vi "Build Command.vi"(8 "error in":errorcluster, 9 "Input Value":string, 10 "Commands":T1, 11 "ESM303 in":refnum<class "ESM303.lvclass">) -> (0 "error out":errorcluster, 1 "Response Expected?":bool, 2 "Command":string, 3 "ESM303 out":refnum<class "ESM303.lvclass">)   [LabVIEW 2018, in "ESM303.lvlib" / "ESM303.lvclass"]
uses:
  ESM303.lvclass
  builds/Force Test Stand.lvlibp/Custom Controls/Commands.ctl
  <vilib>/regexp/Match Regular Expression.xnode
  builds/Force Test Stand.lvlibp/Force Test Stand.lvclass
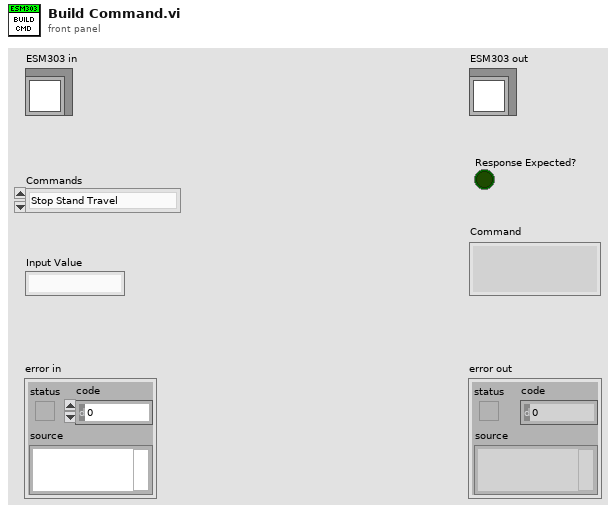
[diagram p1: front panel]
types:
  T1 = typedef "Force Test Stand.lvlibp/Force Test Stand.lvclass/Commands.ctl" = enum16{"Stop Stand Travel", "Start Travel Down (Left)", "Start Travel Up (Right)", "Get Travel Upper Limit", "Get Travel Lower Limit", "Set Travel Upper Limit", "Set Travel Lower Limit", "Get Travel Value", "Set Travel Units (mm)", "Set Travel Units (in)", "Reset Travel to Zero", "Get Speed ", "Set Speed", "Set Speed to Min", "Set Speed to Max", "Get Force Value", "Get Force Units", "Set Force Units (lbF)", "Get Stand Status", "Set Cycle Mode", "Set Limit Mode", "Set Manual Mode", "Set No. Cycles", "Get Travel/Force Values", "Get Completed Cycles", "Get Cycles Setpoint", "Reset Cycles Counter", "Zero Force Gauge", "Set Force Upper Limit", "Set Force Lower Limit", "Get Travel Units", "Get Speed Units", "Default", "Set Force Units (N)", "Set Force Units (kgF)", "Set Force Units (ozF)", "Set Force Units (gF)", "Set Force Real Time Mode", "Set Force Peak Tension Mode", "Set Force Peak Compression Mode", "Set Force High Set-Point", "Set Force Low Set-Point", "Gauge Transmit with Units", "Gauge Transmit w/o Units", "Get Peak Compression Force", "Get Peak Tension Force", "Get Real Time Force", "Disable Force High Limit", "Disable Force Low Limit", "Send Speed Setting to Stand"}
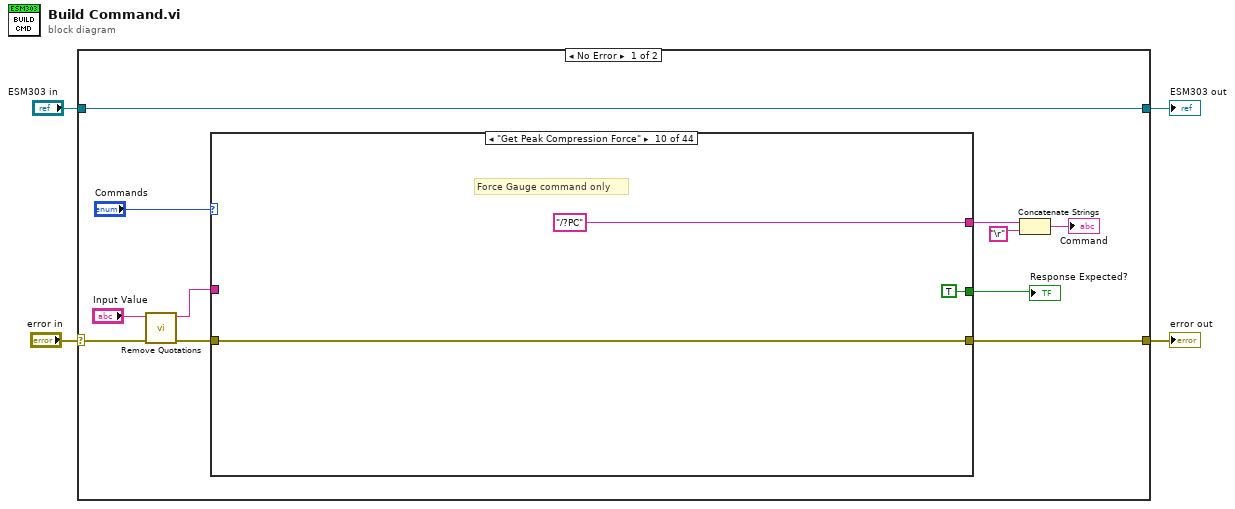
[diagram p0: block diagram]
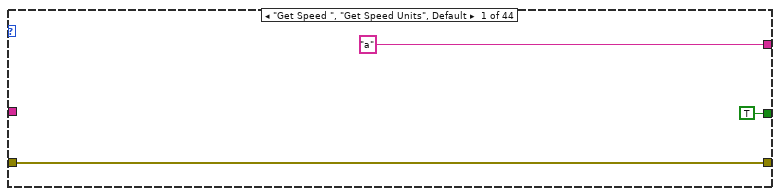
[diagram p2: hidden frame]
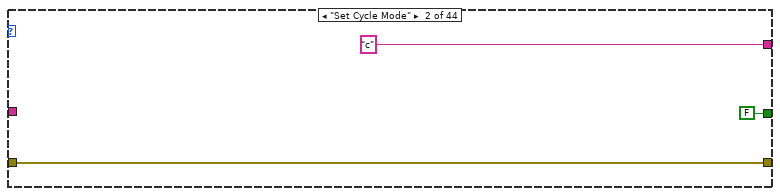
[diagram p3: hidden frame]
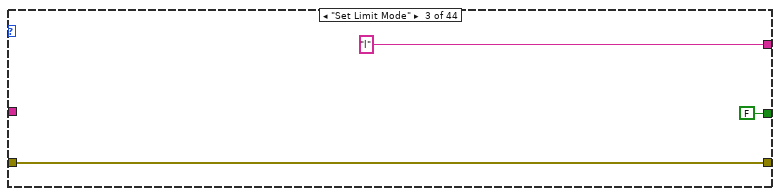
[diagram p4: hidden frame]
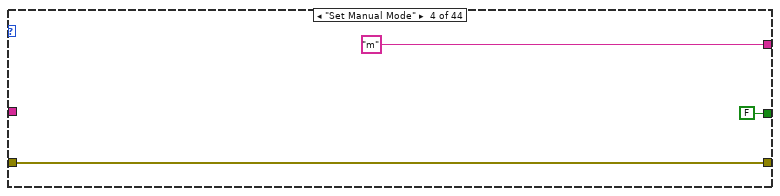
[diagram p5: hidden frame]
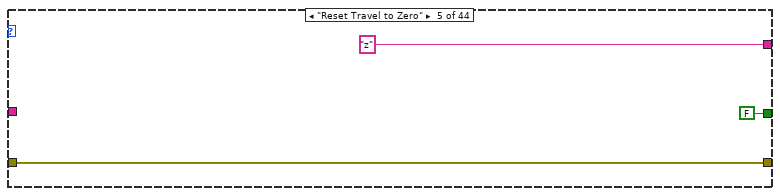
[diagram p6: hidden frame]
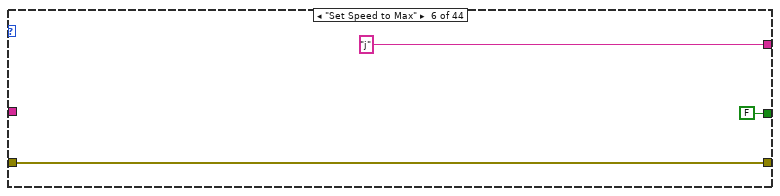
[diagram p7: hidden frame]
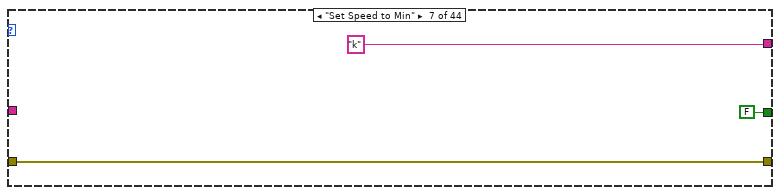
[diagram p8: hidden frame]
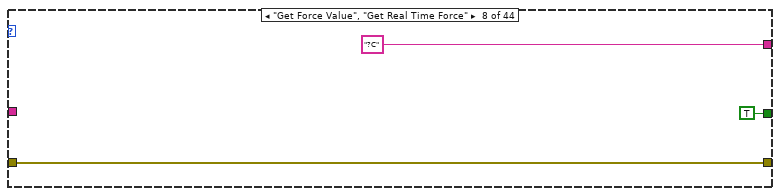
[diagram p9: hidden frame]
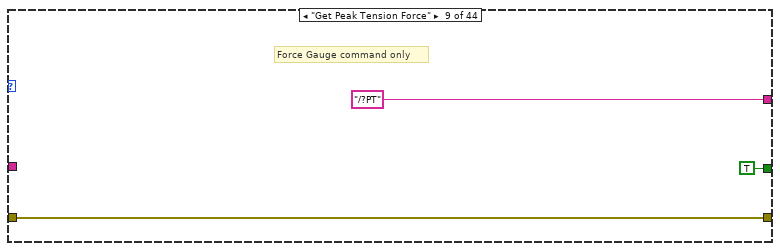
[diagram p10: hidden frame]
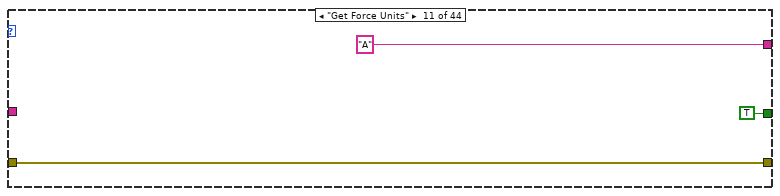
[diagram p11: hidden frame]
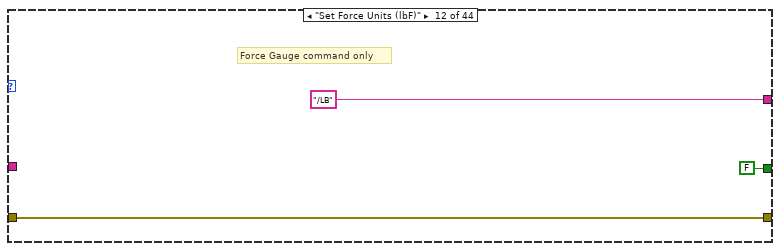
[diagram p12: hidden frame]
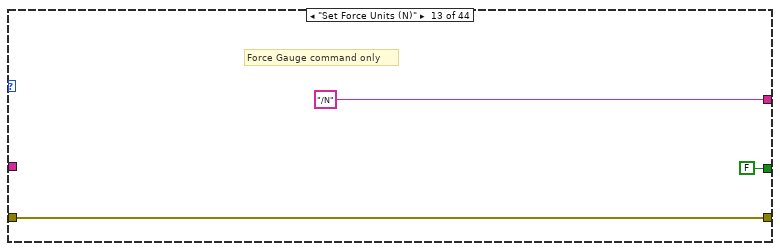
[diagram p13: hidden frame]
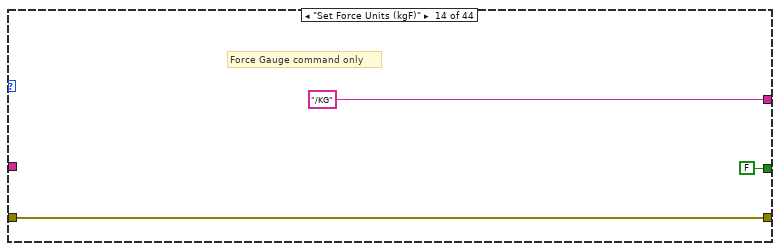
[diagram p14: hidden frame]
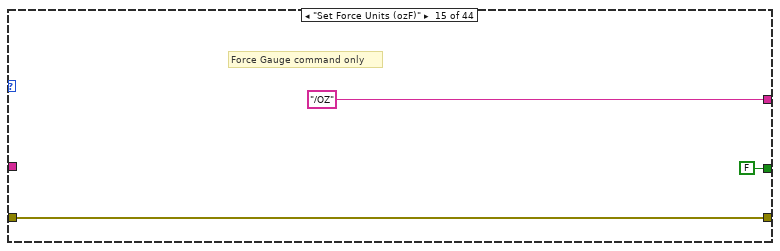
[diagram p15: hidden frame]
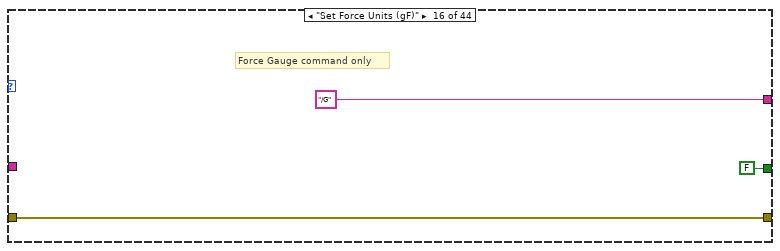
[diagram p16: hidden frame]
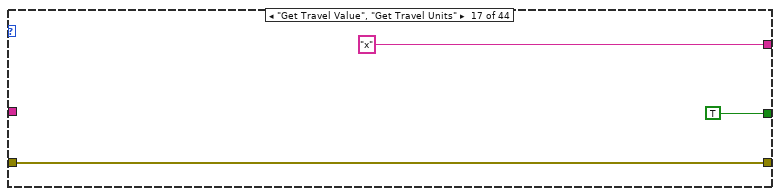
[diagram p17: hidden frame]
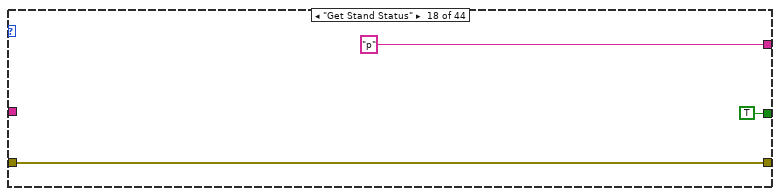
[diagram p18: hidden frame]
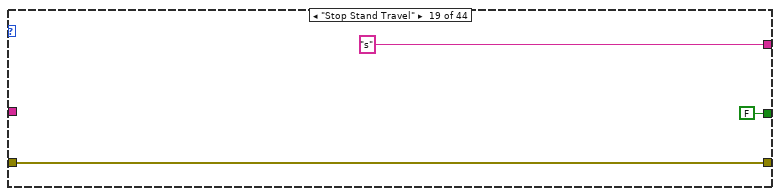
[diagram p19: hidden frame]
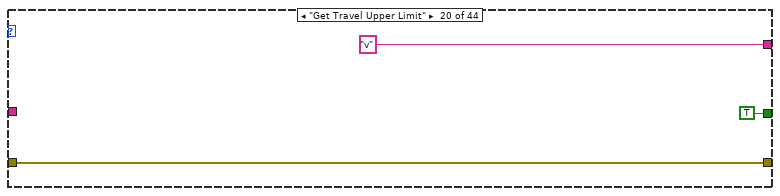
[diagram p20: hidden frame]
diagram:
  n1 = case shown="No Error" "error in" {
    selector: "error in" -> [w8 w549]
    tunnel: [w13 w549] -> w3
    tunnel: [w15 w548] -> w1
    tunnel: "ESM303 in" -> [w15 w548]
    frame No Error {
      n2 = call "Remove Quotations.vi"("error in (no error)"=w8, "With Quotations"="Input Value") -> ("error out"=w5:errorcluster, "Without Quotations"=w6:string)  [unwired: 8 in]
      n3 = case shown="\"Get Peak Compression Force\"" "Commands" {
        selector: "Commands" -> [_ _ _ _ _ _ _ _ _ _ _ _ _ _ _ _ _ _ _ _ _ _ _ _ _ _ w225 _ _ _ _ _ _ _ _ _ _ _ _ _ _ _ _ _]
        tunnel: w5 -> [w17 w20 w23 w26 w29 w32 w36 w39 w42 w45 w48 w51 w54 w57 w60 w63 w65 w68 w71 w74 w77 w80 w83 w87 w90 w92 w226 w362 w490 w493 w496 w499 w502 w504 w507 w510 w516 w521 w526 w531 w536 w541 w544 w547]
        tunnel: w6 -> [_ _ _ _ _ _ _ _ _ _ _ _ _ _ _ _ _ _ _ _ _ _ _ _ _ w98 w222 w364 _ _ _ _ _ _ _ _ w514 w519 w524 w529 w534 _ _ _]
        tunnel: ["a" "c" "l" "m" "z" "j" "k" "?C" "/?PT" "/?PC" "A" "/LB" "/N" "/KG" "/OZ" "/G" "x" "p" "s" "v" "w" "d" "u" "b" "i" w100 w232 w357 "n" "q" "r" "t" "R" "/CUR" "/PT" "/PC" w513 w518 w523 w528 w533 "/SPHD" ("Input Value") "/SPLD" ("Input Value") "o" ("Input Value")] -> w12
        tunnel: [w17 w20 w23 w26 w29 w32 w36 w39 w42 w45 w48 w51 w54 w57 w60 w63 w65 w68 w71 w74 w77 w80 w83 w87 w90 w93 w227 w361 w490 w493 w496 w499 w502 w504 w507 w510 w516 w521 w526 w531 w536 w541 w544 w547] -> w13
        tunnel: [TRUE FALSE FALSE FALSE FALSE FALSE FALSE TRUE TRUE TRUE TRUE FALSE FALSE FALSE FALSE FALSE TRUE TRUE FALSE TRUE TRUE FALSE FALSE FALSE FALSE FALSE FALSE FALSE TRUE TRUE TRUE FALSE FALSE FALSE FALSE FALSE FALSE FALSE FALSE FALSE FALSE FALSE FALSE FALSE] -> w9
        frame "Get Speed ", "Get Speed Units", Default {
        }
        frame "Set Cycle Mode" {
        }
        frame "Set Limit Mode" {
        }
        frame "Set Manual Mode" {
        }
        frame "Reset Travel to Zero" {
        }
        frame "Set Speed to Max" {
        }
        frame "Set Speed to Min" {
        }
        frame "Get Force Value", "Get Real Time Force" {
        }
        frame "Get Peak Tension Force" {
          # "Force Gauge command only"
        }
        frame "Get Peak Compression Force" {
          # "Force Gauge command only"
        }
        frame "Get Force Units" {
        }
        frame "Set Force Units (lbF)" {
          # "Force Gauge command only"
        }
        frame "Set Force Units (N)" {
          # "Force Gauge command only"
        }
        frame "Set Force Units (kgF)" {
          # "Force Gauge command only"
        }
        frame "Set Force Units (ozF)" {
          # "Force Gauge command only"
        }
        frame "Set Force Units (gF)" {
          # "Force Gauge command only"
        }
        frame "Get Travel Value", "Get Travel Units" {
        }
        frame "Get Stand Status" {
        }
        frame "Stop Stand Travel" {
        }
        frame "Get Travel Upper Limit" {
        }
        frame "Get Travel Lower Limit" {
        }
        frame "Start Travel Down (Left)" {
          # "use also for moving the stand left."
        }
        frame "Start Travel Up (Right)" {
          # "use also to move the stand right."
        }
        frame "Set Travel Units (in)" {
        }
        frame "Set Travel Units (mm)" {
        }
        frame "Set Speed" {
          # "Reg Expression checks for XX.XX or XXXX.X format"
          n4 = xnode "Match Regular Expression"("input string"=w98, "regular expression"="^([0-9][0-9][.][0-9][0-9]|[0-9][0-9][0-9][0-9][.][0-9])$") -> ("whole match"=w95:string, "offset past match"=w96:i32)  [unwired: 4 in, 3 out]
          n5 = case shown="5, 6" w96 {
            tunnel: w95 -> [_ w107]
            tunnel: [_ w107] -> w94
            tunnel: [w104 w106] -> w93
            tunnel: w92 -> [w105 w106]
            frame Default {
              n6 = Bundle By Name(cluster=w105, "status"=TRUE, "code"=9999, "source"="The speed format from in the 'Set Speed' case from \"Build Command.vi\" was  ill-formed. Format expected in Input Value control is XX.XX for in/min or XXXX.X for mm/min.") -> (w104:errorcluster)
            }
            frame 5, 6 {
              # "5: XX.XX in/min\n6: XXXX.X mm/min"
            }
          }
          n7 = Concatenate Strings("e", w94) -> (w100:string)
        }
        frame "Set Travel Upper Limit", "Set Travel Lower Limit" {
          # "Reg Expression checks for +/-XX.XX or +/-XXX.XX format"
          n8 = xnode "Match Regular Expression"("input string"=w222, "regular expression"="^([-]?[0-9][0-9][.][0-9][0-9][0-9]|[-]?[0-9][0-9][0-9][.][0-9][0-9])$") -> ("whole match"=w229:string, "offset past match"=w230:i32)  [unwired: 4 in, 3 out]
          n9 = case shown="Default" w225 {
            tunnel: ["h" _ "g"] -> w224
            frame "Set Travel Upper Limit" {
            }
            frame Default {
            }
            frame "Set Travel Lower Limit" {
            }
          }
          n10 = case shown="Default" w230 {
            tunnel: w229 -> [_ w241]
            tunnel: [_ w241] -> w228
            tunnel: [w238 w240] -> w227
            tunnel: w226 -> [w239 w240]
            frame Default {
              n11 = Bundle By Name(cluster=w239, "status"=TRUE, "code"=9999, "source"="Input Value control for setting the Lower/Upper Travel Limit from Build Command.vi was ill-formed.") -> (w238:errorcluster)
            }
            frame 6, 7 {
            }
          }
          n12 = Concatenate Strings(w224, w228) -> (w232:string)
        }
        frame "Set No. Cycles" {
          # "Reg Expression checks for XXXX  format"
          n13 = xnode "Match Regular Expression"("input string"=w364, "regular expression"="^([0-9][0-9][0-9][0-9])$") -> ("whole match"=w360:string, "offset past match"=w363:i32)  [unwired: 4 in, 3 out]
          n14 = case shown="4" w363 {
            tunnel: w362 -> [w367 w373]
            tunnel: [w366 w373] -> w361
            tunnel: w360 -> [w371 w372]
            tunnel: [w371 w372] -> w358
            frame Default {
              n15 = Bundle By Name(cluster=w367, "status"=TRUE, "code"=9999, "source"="Input Value control for Number of Cycles from Build Command.vi was ill-formed.") -> (w366:errorcluster)
            }
            frame 4 {
            }
          }
          n16 = Concatenate Strings("f" ("string"), w358) -> (w357:string)
        }
        frame "Get Travel/Force Values" {
        }
        frame "Get Completed Cycles" {
        }
        frame "Get Cycles Setpoint" {
        }
        frame "Reset Cycles Counter" {
        }
        frame "Zero Force Gauge" {
        }
        frame "Set Force Real Time Mode" {
          # "Force Gauge command only"
        }
        frame "Set Force Peak Tension Mode" {
          # "Force Gauge command only"
        }
        frame "Set Force Peak Compression Mode" {
          # "Force Gauge command only"
        }
        frame "Set Force High Set-Point" {
          # "Force Gauge command only"
          n17 = Concatenate Strings("/SPH", w514) -> (w513:string)
        }
        frame "Set Force Low Set-Point" {
          # "Force Gauge command only"
          n18 = Concatenate Strings("/SPL", w519) -> (w518:string)
        }
        frame "Gauge Transmit with Units" {
          # "Force Gauge command only"
          n19 = Concatenate Strings("/FULL", w524) -> (w523:string)
        }
        frame "Gauge Transmit w/o Units" {
          # "Force Gauge command only"
          n20 = Concatenate Strings("/NUM", w529) -> (w528:string)
        }
        frame "Default" {
          n21 = Empty String/Path?(string/path=w534) -> (empty?=w535:bool)
          n22 = case shown="False" w535 {
            tunnel: w534 -> [w537 _]
            tunnel: [w537 "\\"] -> w533
            frame False {
            }
            frame True {
            }
          }
        }
        frame "Disable Force High Limit" {
        }
        frame "Disable Force Low Limit" {
        }
        frame "Send Speed Setting to Stand" {
        }
      }
      "Response Expected?" <- w9
      n23 = Concatenate Strings(w12, "\r") -> (→"Command":string)
    }
    frame Error {
    }
  }
  "error out" <- w3
  "ESM303 out" <- w1
